vi "Prepare CONNACK Response.vi"(8 "error in (no error)":errorcluster, 9 "Return Code":T1, 10 "Session Present":bool, 11 "CONNECT in":refnum<class "CONNECT.lvclass">) -> (0 "error out":errorcluster, 1 "response prepared?":bool, 2 "CONNACK response":refnum<class "CONNACK.lvclass">, 3 "CONNECT out":refnum<class "CONNECT.lvclass">)   [LabVIEW 2013, in "MQTT_Control_Packets.lvlib" / "CONNECT.lvclass"]
uses:
  CONNECT.lvclass
  CONNACK/CONNACK.lvclass
  CONNACK/Connect Return Code -- enum.ctl
  ControlPacket/ControlPacket.lvclass/ControlPacket.ctl
  ControlPacket/ControlPacket.lvclass
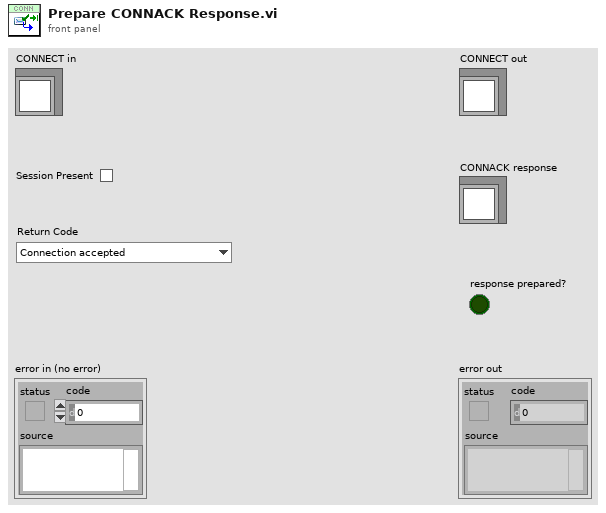
[diagram p1: front panel]
types:
  T1 = typedef "MQTT_Control_Packets.lvlib/CONNACK.lvclass/Connect Return Code -- enum.ctl" = enum16{"Connection accepted", "Unacceptable protocol version", "Identifier Rejected", "Server Unavailable", "Bad Username or Password", "Not Authorized"}
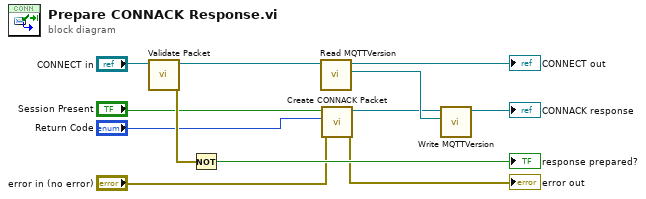
[diagram p0: block diagram]
diagram:
  n1 = call "Validate Packet.vi"("ControlPacket in"="CONNECT in") -> ("error out"=w11:errorcluster, "ControlPacket out"=w10:refnum<class "CONNECT.lvclass">)  [unwired: 9 in]
  n2 = Not(x=w11) -> (.not. x?=→"response prepared?":bool)
  n3 = call "Read MQTTVersion.vi"("ControlPacket in"=w10) -> ("MQTTVersion"=w12:refnum<class "MQTTVersion.lvclass">, "ControlPacket out"=→"CONNECT out":refnum<class "CONNECT.lvclass">)  [unwired: 9 in]
  n4 = call "Create CONNACK Packet.vi"("error in (no error)"="error in (no error)", "Return Code"="Return Code", "Session Present"="Session Present") -> ("error out"=→"error out":errorcluster, "CONNACK"=w7:refnum<class "CONNACK.lvclass">)  [unwired: 6 in, 1 out]
  n5 = call "Write MQTTVersion.vi"("MQTTVersion"=w12, "ControlPacket in"=w7) -> ("ControlPacket out"=→"CONNACK response":refnum<class "CONNACK.lvclass">)  [unwired: 9 in]
